vi "Put Object from RAW data.vi"(7 "Request Parameters":T2={"Content Type"="binary/octet-stream", "ACL"=enum."private", "Storage Class"=enum."STANDARD", "User Metadata"=[], "Content MD5"=""}, 8 "error in (no error)":errorcluster, 9 "Bucket":string, 10 "Path":string, 11 "Data":string) -> (0 "error out":errorcluster, 3 "PutObjectResult":T1)   [LabVIEW 2011, in "LV Interface for Amazon S3.lvlib"]
doc: "This operation <B>adds an object to a bucket</B>. You <B>must have WRITE permissions on a bucket</B> to add an object to it. Amazon S3 <B>never adds partial objects</B>; if you receive no error response, Amazon S3 added the entire object to the bucket. Amazon S3 is a distributed system. If Amazon S3 receives multiple write requests for the same object simultaneously, all but the last object written will be overwritten. Amazon S3 does not provide object locking; if you need this, make sure to build it into your application layer or use versioning instead."
uses:
  LV Interface for Amazon S3.lvlib
  Typedefs/AMZ_S3_API_PUT Object Request Parameters.ctl
  Typedefs/AMZ_S3_ACL.ctl
  Typedefs/AMZ_S3_Storage Class.ctl
  Typedefs/AMZ_S3_Object Metadata.ctl
  Typedefs/AMZ_S3_API_PUTObjectResult.ctl
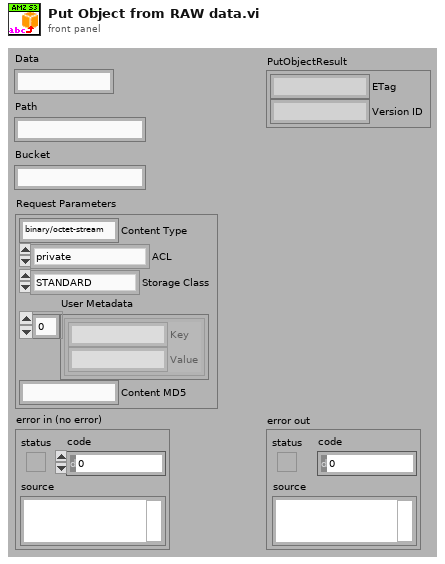
[diagram p1: front panel]
types:
  T1 = typedef "LV Interface for Amazon S3.lvlib/AMZ_S3_API_PUTObjectResult.ctl" = cluster{"ETag":string, "Version ID":string}
  T2 = typedef "LV Interface for Amazon S3.lvlib/AMZ_S3_API_PUT Object Request Parameters.ctl" = cluster{"Content Type":string, "ACL":T3, "Storage Class":T4, "User Metadata":T5[], "Content MD5":string}
  T3 = typedef "LV Interface for Amazon S3.lvlib/AMZ_S3_ACL.ctl" = enum16{"private", "public-read", "public-read-write", "authenticated-read", "bucket-owner-read", "bucket-owner-full-control"}
  T4 = typedef "LV Interface for Amazon S3.lvlib/AMZ_S3_Storage Class.ctl" = enum16{"STANDARD", "REDUCED_REDUNDANCY"}
  T5 = typedef "LV Interface for Amazon S3.lvlib/AMZ_S3_Object Metadata.ctl" = cluster{"Key":string, "Value":string}
  T6 = typedef "LV Interface for Amazon S3.lvlib/AMZ_S3_HTTP Header-Value pair.ctl" = cluster{"Header":string, "Value":string}
  T7 = typedef "LV Interface for Amazon S3.lvlib/AMZ_S3_Call Results.ctl" = enum16{"Success", "UndefinedError", "AccessDenied", "AccountProblem", "AmbiguousGrantByEmailAddress", "BadDigest", "BucketAlreadyExists", "BucketAlreadyOwnedByYou", "BucketNotEmpty", "CredentialsNotSupported", "CrossLocationLoggingProhibited", "EntityTooSmall", "EntityTooLarge", "ExpiredToken", "IllegalVersioningConfigurationException", "IncompleteBody", "IncorrectNumberOfFilesInPostRequest", "InlineDataTooLarge", "InternalError", "InvalidAccessKeyId", "InvalidAddressingHeader", "InvalidArgument", "InvalidBucketName", "InvalidDigest", "InvalidLocationConstraint", "InvalidPart", "InvalidPartOrder", "InvalidPayer", "InvalidPolicyDocument", "InvalidRange", "InvalidSecurity", "InvalidSOAPRequest", "InvalidStorageClass", "InvalidTargetBucketForLogging", "InvalidToken", "InvalidURI", "KeyTooLong", "MalformedACLError", "MalformedPOSTRequest", "MalformedXML", "MaxMessageLengthExceeded", "MaxPostPreDataLengthExceededError", "MetadataTooLarge", "MethodNotAllowed", "MissingAttachment", "MissingContentLength", "MissingRequestBodyError", "MissingSecurityElement", "MissingSecurityHeader", "NoLoggingStatusForKey", "NoSuchBucket", "NoSuchKey", "NoSuchUpload", "NoSuchVersion", "NotImplemented", "NotSignedUp", "OperationAborted", "PermanentRedirect", "PreconditionFailed", "Redirect", "RequestIsNotMultiPartContent", "RequestTimeout", "RequestTimeTooSkewed", "RequestTorrentOfBucketError", "SignatureDoesNotMatch", "SlowDown", "TemporaryRedirect", "TokenRefreshRequired", "TooManyBuckets", "UnexpectedContent", "UnresolvableGrantByEmailAddress", "UserKeyMustBeSpecified", "LabVIEWError"}
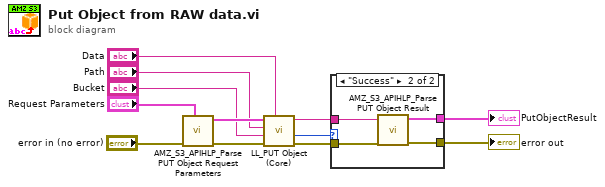
[diagram p0: block diagram]
diagram:
  n1 = call "AMZ_S3_APIHLP_Parse PUT Object Request Parameters.vi"("PUT Object Request Parameters"="Request Parameters", "error in (no error)"="error in (no error)") -> ("error out"=w12:errorcluster, "HTTP Headers"=w11:T6[])  [unwired: 8 in]
  n2 = call "LL_PUT Object (Core).vi"("Data"="Data", "error in (no error)"=w12, "Bucket"="Bucket", "Path and query string"="Path", "Headers"=w11) -> ("error out"=w4:errorcluster, "Call Result"=w5:T7, "Response header"=w3:string)  [unwired: 3 in, 1 out]
  n3 = case shown="\"Success\"" w5 {
    tunnel: w4 -> [w13 w17]
    tunnel: w3 -> [_ w16]
    tunnel: [_ w15] -> w1
    tunnel: [w13 w14] -> w2
    frame Default {
    }
    frame "Success" {
      n4 = call "AMZ_S3_APIHLP_Parse PUT Object Result.vi"("error in (no error)"=w17, "Response header"=w16) -> ("error out"=w14:errorcluster, "PutObjectResult"=w15:T1)  [unwired: 8 in]
    }
  }
  "error out" <- w2
  "PutObjectResult" <- w1
